vi "Simple Read.vi"(4 "Abs_Variant in":refnum<class "Abs_Variant.lvclass">) -> (1 "Variant":variant)   [LabVIEW 2021, in "Abs_Variant.lvclass"]
uses:
  Abs_Variant.lvclass
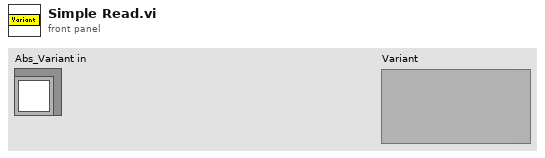
[diagram p1: front panel]
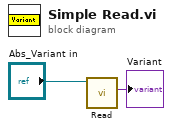
[diagram p0: block diagram]
diagram:
  n1 = call-dynamic "Read.vi"("Abs_Variant in"="Abs_Variant in") -> ("Variant"=→"Variant":variant)  [unwired: 8 in, 2 out]
